vi "BotSpeak_Servo.vi"(0 "Duty (msec)":dbl=1.5, 2 "Bot Settings":T1, 3 "DIO Line":u8(slide) scale=0.0..3.0) -> (4 "Bot Settings 2":T1)   [LabVIEW 2014]
doc: "Runs a servo motor wired to the specified \"DIO Line\" with the specified \"Duty\" time.\n1 ms is all the way in one direction\n2 ms is all the way in the other direction\n1.5 ms is in the middle"
uses:
  <userlib>/BotSpeak/VIs/Direct/BotSpeak_Control.ctl
panel:
  out "response":string
  # "range from 0 to 3 msec"
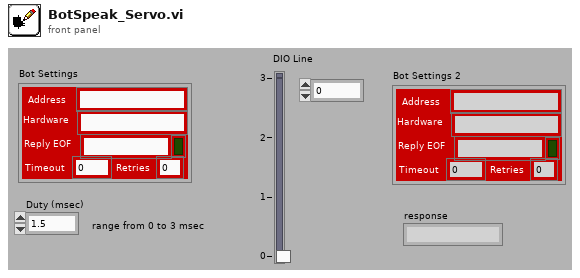
[diagram p1: front panel]
types:
  T1 = typedef "BotSpeak_Control.ctl" = cluster{"Address":string, "Reply EOF":string, "Hardware":string, "Retries":i8, "Timeout":i32, "Open?":bool}
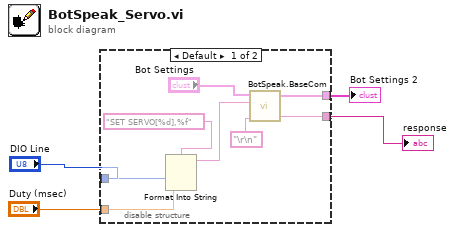
[diagram p0: block diagram]
diagram:
  n1 = disable-structure shown="Default" {
    disable-tunnel: [w9 _] -> w4
    disable-tunnel: [w8 _] -> w3
    disable-tunnel: "DIO Line" -> [w7 _]
    disable-tunnel: "Duty (msec)" -> [w6 _]
    frame condition #0 {
      n2 = Format Into String(format string="SET SERVO[%d],%f" ("command"), w7, w6) -> (resulting string=w12:string)  [unwired: 2 in, 1 out]
      n3 = call <userlib>:"BotSpeak.BaseCom.vi"("Termination"="\r\n", "command"=w12, "Bot Settings in"="Bot Settings") -> ("response"=w8:string, "Bot Settings out"=w9:T1)  [unwired: 2 in]
    }
    frame condition #1 (active) {
    }
  }
  "Bot Settings 2" <- w4
  "response" <- w3
